vi "Build Directory Tree.vi"(3 "Root Directory":string="/", 4 "Directory Tree in":T1, 5 "Printed Data on Terminal":string[](array[string])) -> (1 "Directory Tree out":T1)   [LabVIEW 2020, in "AoC 2022.lvlib"]
uses:
  AoC 2022.lvlib
  Directory Tree.ctl
  Directory Contents.ctl
  File.ctl
  <vilib>/Utility/miscctls.llb/LVMapReplaceAction.ctl
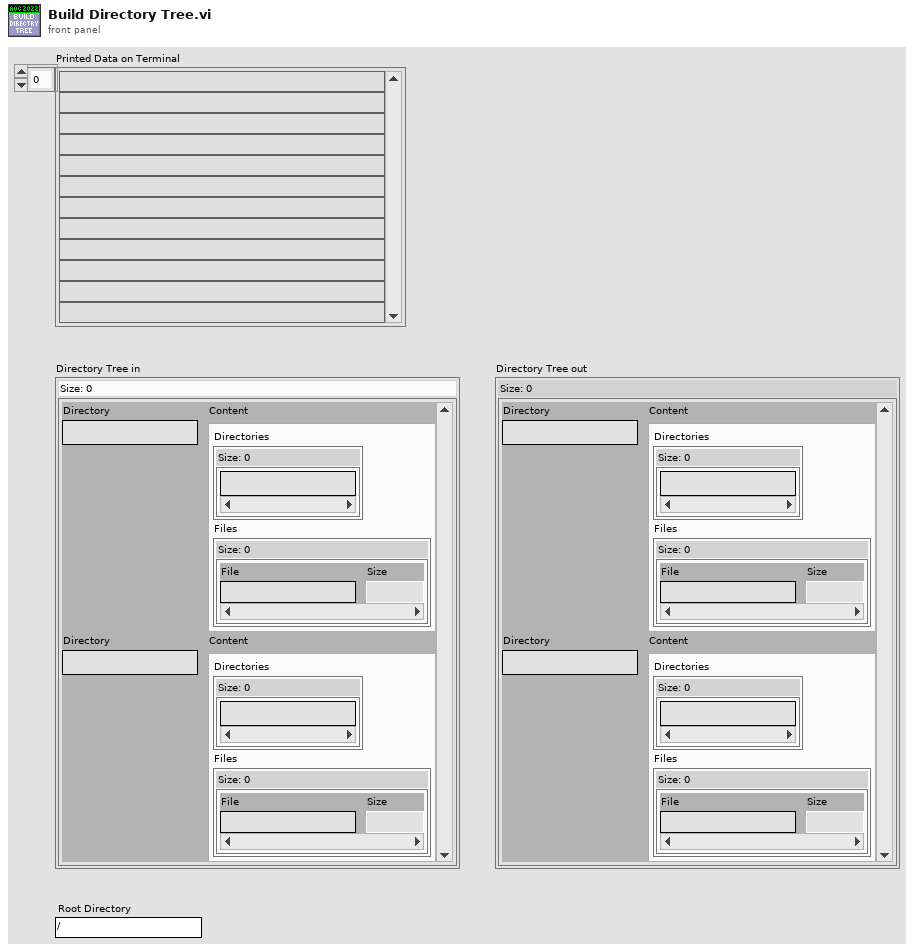
[diagram p1: front panel]
types:
  T1 = typedef "AoC 2022.lvlib/Directory Tree.ctl" = map{string, T2}
  T2 = typedef "AoC 2022.lvlib/Directory Contents.ctl" = cluster{"Directories":set{string}, "Files":T3}
  T3 = typedef "AoC 2022.lvlib/File.ctl" = map{string, u64}
  T4 = typedef "LVMapReplaceAction.ctl" = enum32{"Modify Entry only if found", "Add or Modify Entry", "Delete Entry"}
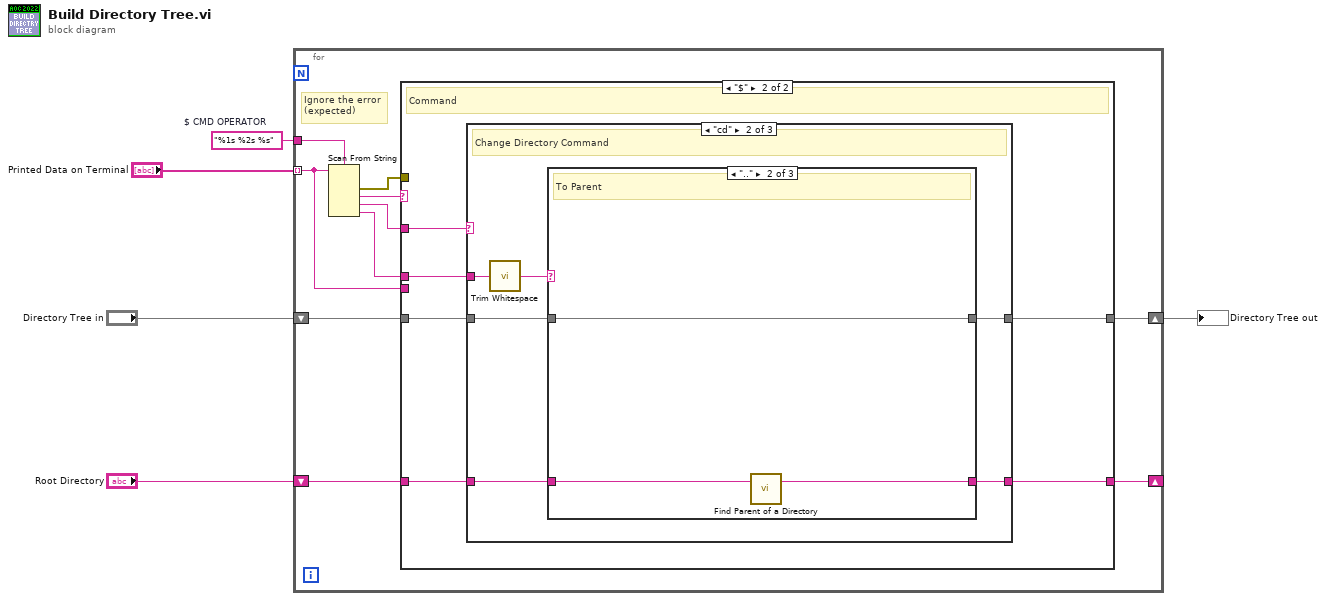
[diagram p0: block diagram]
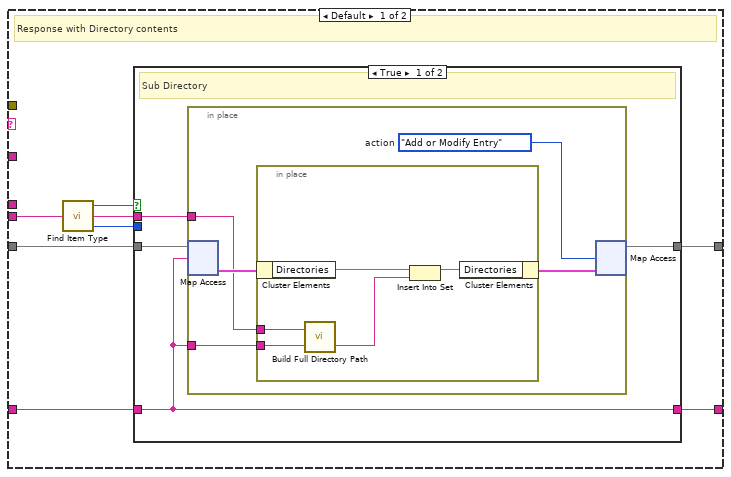
[diagram p2: hidden frame]
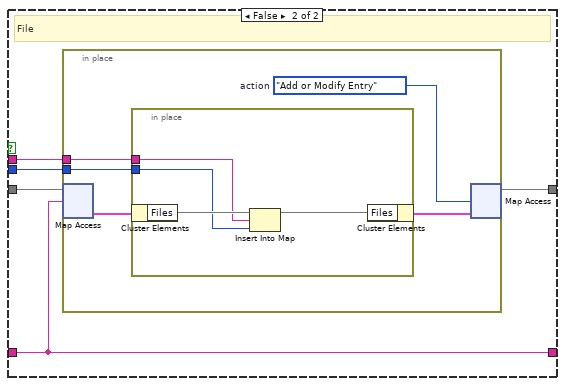
[diagram p3: hidden frame]
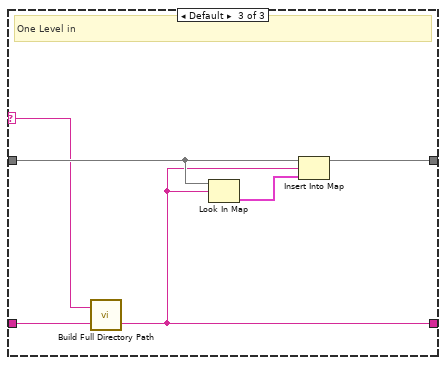
[diagram p6: hidden frame]
diagram:
  w2 = "%1s %2s %s"  # $ CMD OPERATOR
  n1 = for {
    tunnel: "Printed Data on Terminal" -> [w8] mode=indexing
    shift-right: [w13] -> w5
    shift-left: "Directory Tree in" -> [w12]
    tunnel: w2 -> [w15]
    shift-right: [w10] -> _
    shift-left: "Root Directory" -> [w11]
    # "Ignore the error\n(expected)"
    n2 = Scan From String(format string=w15, input string=w8) -> (error out=w9:errorcluster, output 1=w14:string, output 2=w7:string, output 3=w6:string)  [unwired: 5 in, 2 out]
    n3 = case shown="\"$\"" w14 {
      tunnel: w7 -> [_ w57]
      tunnel: [w17 w56] -> w13
      tunnel: w12 -> [w22 w55]
      tunnel: w11 -> [w18 w54]
      tunnel: w6 -> [_ w53]
      tunnel: [w16 w52] -> w10
      tunnel: w9 -> [_ _]
      tunnel: w8 -> [w23 _]
      frame Default {
        # "Response with Directory contents"
        n4 = call "Find Item Type.vi"("Directory Item in"=w23) -> ("Directory?"=w21:bool, "Item Name"=w20:string, "Item Size"=w19:u64)
        n5 = case shown="True" w21 {
          tunnel: w22 -> [w27 w42]
          tunnel: w20 -> [w25 w39]
          tunnel: w19 -> [_ w38]
          tunnel: w18 -> [w24 w40]
          tunnel: [w26 w41] -> w17
          tunnel: [w24 w40] -> w16
          frame True {
            # "Sub Directory"
            n6 = in-place {
              in-place-border: w25 -> [w28]
              in-place-border: w24 -> [w29]
              w30 = LVMapReplaceAction."Add or Modify Entry"  # action
              n7 = in-place-map #1(w27, w24) -> (w32:T2)  [unwired: 1 in, 1 out]
              n8 = in-place {
                in-place-border: w29 -> [w35]
                in-place-border: w28 -> [w33]
                n9 = in-place-cluster #2(w32) -> ("Directories"=w37:set{string})
                n10 = call "Build Full Directory Path.vi"("Parent Directory"=w35, "Sub Directory"=w33) -> ("Full Directory Path"=w34:string)  [unwired: 1 in]
                n11 = Insert Into Set(10:w34, 11:w37) -> (3:w36:set{string})  [unwired: 1 out]
                n12 = in-place-cluster #2("Directories"=w36) -> (w31:T2)
              }
              n13 = in-place-map #1(w31, w30) -> (w26:T1)  [unwired: 2 out]
            }
          }
          frame False {
            # "File"
            n14 = in-place {
              in-place-border: w39 -> [w44]
              in-place-border: w38 -> [w43]
              w45 = LVMapReplaceAction."Add or Modify Entry"  # action
              n15 = in-place-map #3(w42, w40) -> (w47:T2)  [unwired: 1 in, 1 out]
              n16 = in-place {
                in-place-border: w44 -> [w48]
                in-place-border: w43 -> [w49]
                n17 = in-place-cluster #4(w47) -> ("Files"=w51:T3)
                n18 = Insert Into Map(map in=w51, key=w48, value=w49) -> (map out=w50:T3)  [unwired: 2 out]
                n19 = in-place-cluster #4("Files"=w50) -> (w46:T2)
              }
              n20 = in-place-map #3(w46, w45) -> (w41:T1)  [unwired: 2 out]
            }
          }
        }
      }
      frame "$" {
        # "Command"
        n21 = case shown="\"cd\"" w57 {
          tunnel: [w59 w63 w78] -> w56
          tunnel: w55 -> [w59 w64 w78]
          tunnel: w54 -> [w58 w61 w77]
          tunnel: w53 -> [_ w65 _]
          tunnel: [w58 w60 w77] -> w52
          frame Default {
            # "Unknown command"
          }
          frame "cd" {
            # "Change Directory Command"
            n22 = call <vilib>:"Trim Whitespace.vi"("string"=w65) -> ("trimmed string"=w62:string)  [unwired: 1 in]
            n23 = case shown="\"..\"" w62 {
              selector: w62 -> [w67 _ w72]
              tunnel: w64 -> [w66 w69 w75]
              tunnel: [w66 w69 w76] -> w63
              tunnel: w61 -> [_ w68 w73]
              tunnel: [w67 w70 w71] -> w60
              frame "/" {
                # "Root"
              }
              frame ".." {
                # "To Parent"
                n24 = call "Find Parent of a Directory.vi"("Directory"=w68) -> ("Parent Directory"=w70:string)  [unwired: 1 in, 1 out]
              }
              frame Default {
                # "One Level in"
                n25 = call "Build Full Directory Path.vi"("Parent Directory"=w73, "Sub Directory"=w72) -> ("Full Directory Path"=w71:string)  [unwired: 1 in]
                n26 = Look In Map(map=w75, key=w71) -> (value=w74:T2)  [unwired: 1 in, 1 out]
                n27 = Insert Into Map(map in=w75, key=w71, value=w74) -> (map out=w76:T1)  [unwired: 2 out]
              }
            }
          }
          frame "ls" {
            # "ls - List command"
          }
        }
      }
    }
  }
  "Directory Tree out" <- w5
